vi "GUI TWM setup.vi"(11 "TWM pipe":string="\\\\.\\pipe\\TWM:server") -> (3 "TWM pipe out":string)   [LabVIEW 2020]
doc: "Use this template to build a producer/consumer design pattern with events to produce queue items. Use this design pattern instead of the User Interface Event Handler pattern for user interfaces when you want to execute code asynchronously in response to an event without slowing the user interface responsiveness."
uses:
  <vilib>/Utility/error.llb/DialogType.ctl
  <vilib>/Utility/error.llb/Error Cluster From Error Code.vi
  <vilib>/ErrorRing/Error Ring.xnode
  external libraries/varilib/varilib.lvlib
  external libraries/TWM-1.8.7.0-client/TWM Client.lvlib
panel:
  out "gui_elements":refnum<vi>[](array[refnum])
  out "Status":string
  in  "save_and_quit":bool
  in  "test":bool
  in  "cancel":bool
  # "FF Meter changes following in the TWM:\n1, Sampling rate (TWM->Setup Measurement)\n2, Samples count (TWM->Setup Measurement)\n3, Records count (TWM->Setup Measurement)\n4, Sub-records count (TWM->Setup Measurement)\n5, Trigger (mode, source, level, coupling\n                                     (TWM->Setup Measurment)\n6, Measurement name (TWM->Setup Measurement)\n7, Processing setup"
  # "You must set following in TWM according your setup:\n1, Octave/Matlab\n2, Digitizers"
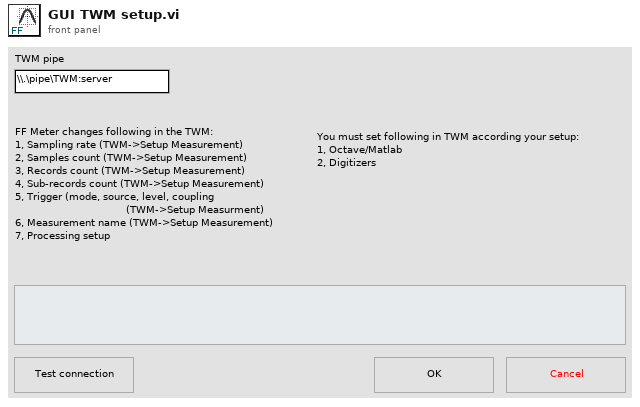
[diagram p1: front panel]
types:
  T1 = typedef "DialogType.ctl" = u16
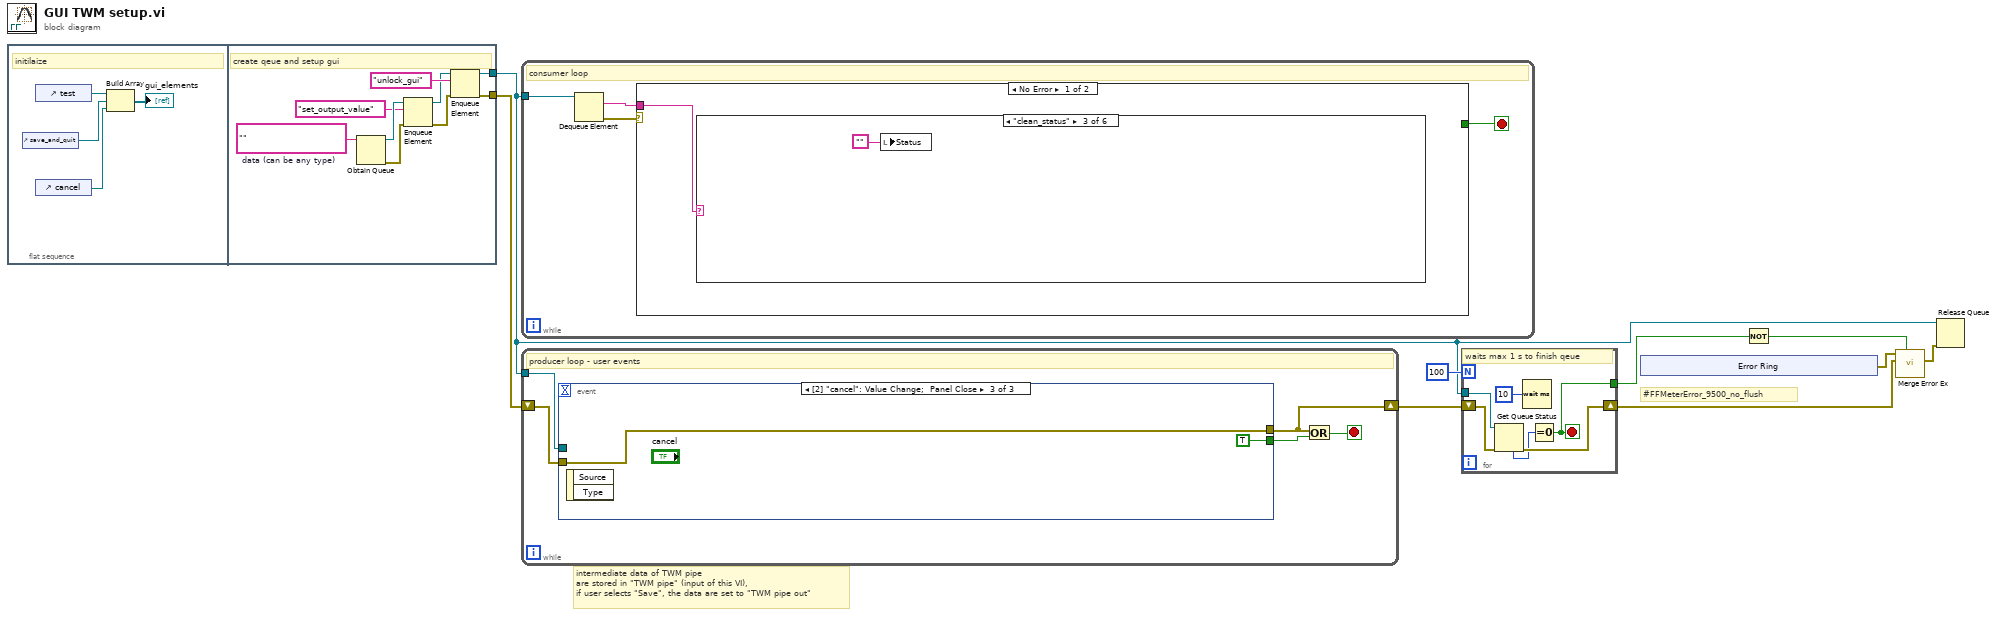
[diagram p0: block diagram]
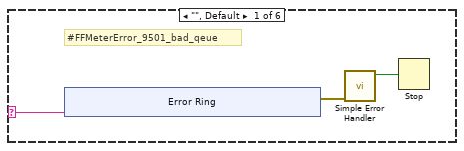
[diagram p2: hidden frame]
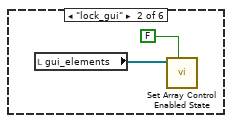
[diagram p3: hidden frame]
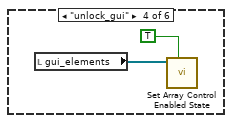
[diagram p4: hidden frame]
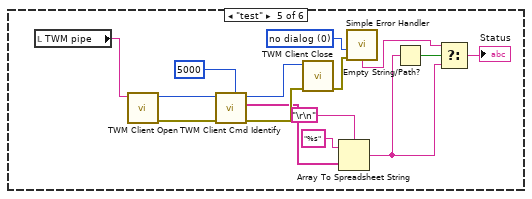
[diagram p5: hidden frame]
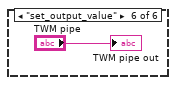
[diagram p6: hidden frame]
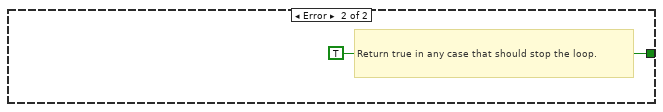
[diagram p7: hidden frame]
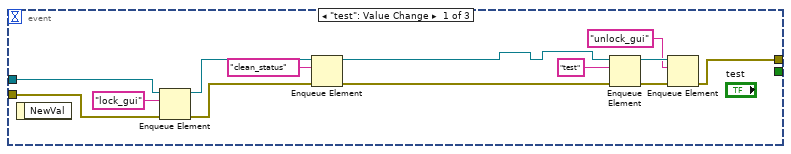
[diagram p8: hidden frame]
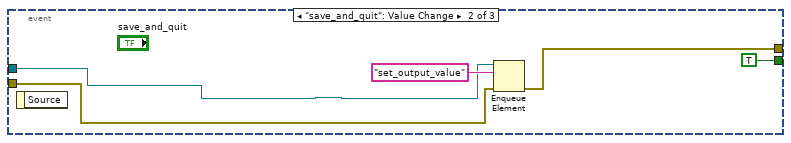
[diagram p9: hidden frame]
diagram:
  # "#FFMeterError_9500_no_flush"
  # "intermediate data of TWM pipe\nare stored in \"TWM pipe\" (input of this VI),\nif user selects \"Save\", the data are set to \"TWM pipe out\""
  n1 = flat-sequence {
    tunnel: [w18] -> w2
    tunnel: [w16] -> w1
    frame #0 {
      # "initilaize"
      n2 = control-ref of="save_and_quit"() -> (w12:refnum<vi>)
      n3 = control-ref of="test"() -> (w13:refnum<vi>)
      n4 = control-ref of="cancel"() -> (w11:refnum<vi>)
      n5 = Build Array(w13, w12, w11) -> (→"gui_elements":refnum<vi>[])
    }
    frame #1 {
      w17 = ""  # data (can be any type)
      # "create qeue and setup gui"
      n6 = Obtain Queue(element data type=w17) -> (queue out=w21:refnum<queue>, error out=w22:errorcluster)  [unwired: 4 in, 1 out]
      n7 = Enqueue Element(queue=w21, element="set_output_value", error in (no error)=w22) -> (queue out=w14:refnum<queue>, error out=w15:errorcluster)  [unwired: 1 in, 1 out]
      n8 = Enqueue Element(queue=w14, element="unlock_gui", error in (no error)=w15) -> (queue out=w18:refnum<queue>, error out=w16:errorcluster)  [unwired: 1 in, 1 out]
    }
  }
  n9 = while {
    tunnel: w2 -> [w26]
    stop <- w23 stop-if-true
    # "consumer loop"
    n10 = Dequeue Element(queue=w26) -> (element=w24:string, error out=w25:errorcluster)  [unwired: 2 in, 2 out]
    n11 = case shown="No Error" w25 {
      tunnel: w24 -> [w27 _]
      tunnel: [_ TRUE] -> w23
      frame No Error {
        n12 = case shown="\"clean_status\"" w27 {
          selector: w27 -> [w28 _ _ _ _ _]
          frame "", Default {
            # "#FFMeterError_9501_bad_qeue"
            n13 = xnode "Error Ring"("parameter 0"=w28) -> ("error out"=w30:errorcluster)
            n14 = call <vilib>:"Simple Error Handler.vi"("error in (no error)"=w30) -> ("error?"=w29:bool)  [unwired: 4 in, 4 out]
            n15 = Stop(stop? (T)=w29) -> ()
          }
          frame "lock_gui" {
            n16 = local read "gui_elements"() -> (w39:refnum<vi>[])
            n17 = call "Set Array Control Enabled State.vi"("enabled (T)"=FALSE, "reference array in"=w39) -> ()  [unwired: 8 in, 2 out]
          }
          frame "clean_status" {
            n18 = local write "Status"("") -> ()
          }
          frame "unlock_gui" {
            n19 = local read "gui_elements"() -> (w42:refnum<vi>[])
            n20 = call "Set Array Control Enabled State.vi"("enabled (T)"=TRUE, "reference array in"=w42) -> ()  [unwired: 8 in, 2 out]
          }
          frame "test" {
            w48 = T1 0 items=["no dialog", "OK message", "continue or stop message", "OK message + warnings", "continue/stop + warnings"] ("type of dialog (OK msg:1)")
            n21 = local read "TWM pipe"() -> (w44:string)
            n22 = call "TWM Client Open.vi"("pipe name"=w44) -> ("error out"=w56:errorcluster, "handle out"=w55:i32)  [unwired: 9 in]
            n23 = call "TWM Client Cmd Identify.vi"("timeout [ms]"=5000, "error in"=w56, "handle"=w55) -> ("error out"=w57:errorcluster, "channel idns"=w52:string[], "handle out"=w54:i32)  [unwired: 5 in, 1 out]
            n24 = call "TWM Client Close.vi"("error in"=w57, "handle in"=w54) -> ("error out"=w49:errorcluster)  [unwired: 9 in]
            n25 = Array To Spreadsheet String(delimiter (Tab)="\r\n", array=w52, 3:"%s" ("format string")) -> (spreadsheet string=w45:string)
            n26 = call <vilib>:"Simple Error Handler.vi"("type of dialog (OK msg:1)"=w48, "error in (no error)"=w49) -> ("message"=w46:string)  [unwired: 3 in, 4 out]
            n27 = Empty String/Path?(string/path=w45) -> (empty?=w47:bool)
            n28 = Select(t=w46, s=w47, f=w45) -> (s? t:f=→"Status":string)
          }
          frame "set_output_value" {
            "TWM pipe out" <- "TWM pipe"
          }
        }
      }
      frame Error {
        # "Return true in any case that should stop the loop."
      }
    }
  }
  n29 = while {
    shift-right: [w60] -> w5
    shift-left: w1 -> [w63]
    tunnel: w2 -> [w64]
    stop <- w61 stop-if-true
    # "producer loop - user events"
    n30 = event shown="[2] \"cancel\": Value Change;  Panel Close" {
      selector: _ -> [_ _ _]
      dyn-events: _ -> [_ _ _]
      timeout: _ -> [_ _ _]
      tunnel: w64 -> [w71 w79 _]
      tunnel: w63 -> [w72 w78 w84]
      tunnel: [w75 w80 w84] -> w60
      tunnel: [_ TRUE ("cancel") TRUE ("cancel")] -> w62
      event "test": Value Change {
        n31 = event-data() -> ()  [unwired: 1 in, 1 out]
        n32 = Enqueue Element(queue=w71, element="lock_gui", error in (no error)=w72) -> (queue out=w68:refnum<queue>, error out=w69:errorcluster)  [unwired: 1 in, 1 out]
        n33 = Enqueue Element(queue=w68, element="clean_status", error in (no error)=w69) -> (queue out=w66:refnum<queue>, error out=w65:errorcluster)  [unwired: 1 in, 1 out]
        n34 = Enqueue Element(queue=w66, element="test", error in (no error)=w65) -> (queue out=w74:refnum<queue>, error out=w76:errorcluster)  [unwired: 1 in, 1 out]
        n35 = Enqueue Element(queue=w74, element="unlock_gui", error in (no error)=w76) -> (error out=w75:errorcluster)  [unwired: 1 in, 2 out]
      }
      event "save_and_quit": Value Change {
        n36 = event-data() -> ()  [unwired: 1 in, 1 out]
        n37 = Enqueue Element(queue=w79, element="set_output_value", error in (no error)=w78) -> (error out=w80:errorcluster)  [unwired: 1 in, 2 out]
      }
      event "cancel": Value Change; Panel Close {
        n38 = event-data() -> ()  [unwired: 1 in, 2 out]
      }
    }
    n39 = Or(x=w60, y=w62) -> (x .or. y?=w61:bool)
  }
  n40 = for {
    N: 100 -> [_]
    tunnel: w2 -> [w90]
    shift-right: [w88] -> w6
    shift-left: w5 -> [w89]
    tunnel: [w85] -> w3
    stop <- w85 stop-if-true
    # "waits max 1 s to finish qeue"
    n41 = Get Queue Status(queue=w90, error in (no error)=w89) -> (error out=w88:errorcluster, # elements in queue=w86:i32)  [unwired: 1 in, 6 out]
    n42 = Wait (ms)(milliseconds to wait=u32 10) -> ()  [unwired: 1 out]
    n43 = Equal To 0?(x=w86) -> (x = 0?=w85:bool)
  }
  n44 = xnode "Error Ring"() -> ("error out"=w7:errorcluster)
  n45 = Not(x=w3) -> (.not. x?=w8:bool)
  n46 = call "Merge Error Ex.vi"("Is error? (False)"=w8, "main error in (no error)"=w6, "second error in"=w7) -> ("error out"=w4:errorcluster)  [unwired: 8 in]
  n47 = Release Queue(queue=w2, error in (no error)=w4) -> ()  [unwired: 1 in, 3 out]
